vi "State Sample size test.vi"() -> ()   [LabVIEW 2015, in "LSR Transmission.lvlib"]
uses:
  LSR Transmission.lvlib
  RDS State Tracker/RDS State Tracker.lvlib
panel:
  out "length 3":i32
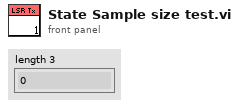
[diagram p1: front panel]
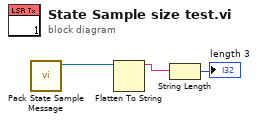
[diagram p0: block diagram]
diagram:
  n1 = call "Pack State Sample Message.vi"() -> ("State Sample Message out"=w1:refnum<class "State Sample Message.lvclass">)  [unwired: 11 in]
  n2 = Flatten To String(anything=w1) -> (data string=w2:string)  [unwired: 3 in, 2 out]
  n3 = String Length(string=w2) -> (length=→"length 3":i32)
